vi "PWM Input Read.vi"(8 "error in (no error)":errorcluster, 11 "NI PWM Input in":refnum<class "NI PWM Input.lvclass">) -> (0 "error out":errorcluster, 2 "Read PWM Data":dbl[][](array[numeric]) format="%0.2f", 3 "NI PWM Input out":refnum<class "NI PWM Input.lvclass">)   [LabVIEW 2023, in "HardwareAbstractionLayer_LVOOP.lvlib" / "NI PWM Input.lvclass"]
uses:
  NI PWM Input.lvclass
  NI PWM Input.lvclass/NI PWM Input.ctl
  <vilib>/DAQmx/read.llb/DAQmx Read (Counter 2D DBL NChan NSamp).vi
  <vilib>/DAQmx/miscellaneous.llb/DAQmx Fill In Error Info.vi
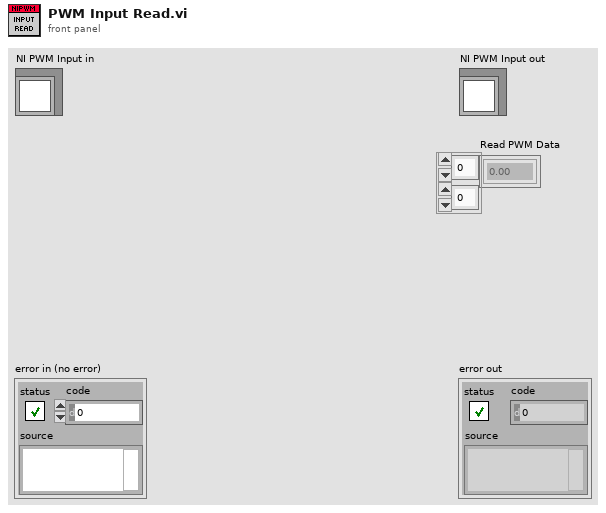
[diagram p1: front panel]
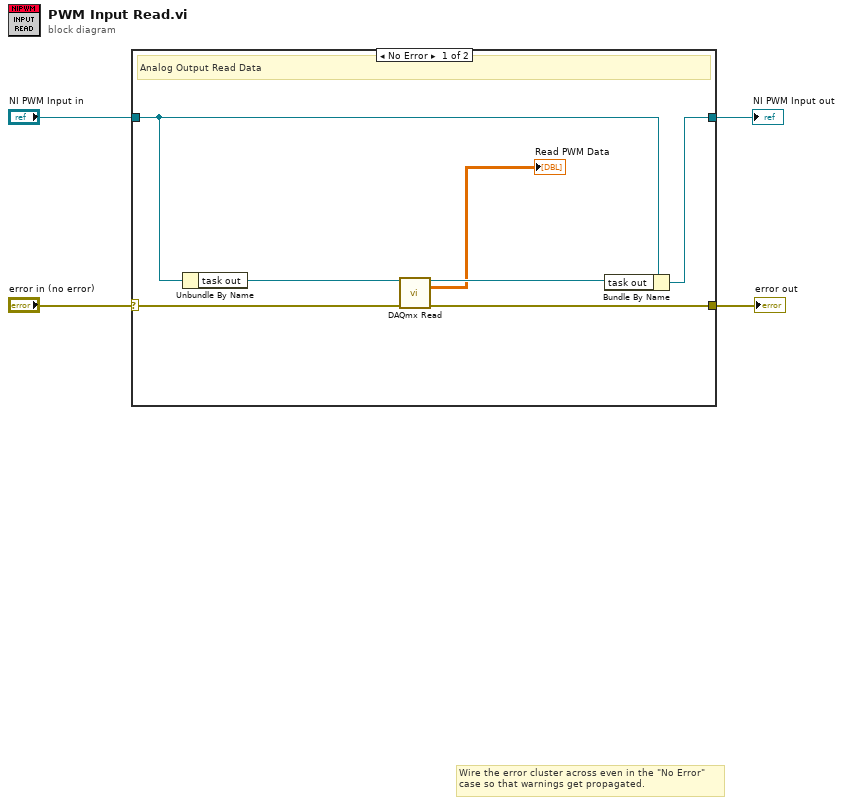
[diagram p0: block diagram]
diagram:
  # "Wire the error cluster across even in the \"No Error\"\ncase so that warnings get propagated."
  n1 = case shown="No Error" "error in (no error)" {
    selector: "error in (no error)" -> [w11 w13]
    tunnel: [w10 w13] -> w3
    tunnel: [w7 w12] -> w1
    tunnel: "NI PWM Input in" -> [w8 w12]
    frame No Error {
      # "Analog Output Read Data"
      n2 = Unbundle By Name(w8) -> ("task out"=w9:refnum<k21>)
      n3 = call-poly <vilib>:"DAQmx Read.vi"("task/channels in"=w9, "error in"=w11) -> ("task out"=w6:refnum<k21>, "data"=→"Read PWM Data":dbl[][], "error out"=w10:errorcluster)  [unwired: 11 in]
      n4 = Bundle By Name(cluster=w8, "task out"=w6) -> (w7:refnum<class "NI PWM Input.lvclass">)
    }
    frame Error {
    }
  }
  "error out" <- w3
  "NI PWM Input out" <- w1
